vi "Change Bit Value.vi"   [LabVIEW 2009, in "IDW.lvlib"]
doc: "Appends a single sample to the I2C waveform wherein one or more of the bus lines (SCL or SDA) changes value."
uses:
  IDW.lvlib
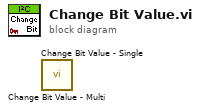
[diagram p0: block diagram]
diagram:
  n1 = call "Change Bit Value - Multi.vi"() -> ()  [unwired: 10 in, 2 out]
  n2 = call "Change Bit Value - Single.vi"() -> ()  [unwired: 10 in, 2 out]
